vi "FGV ErrorLog.vi"(2 "Action":enum16{"Reset", "Enqueue", "Dequeue"}(ring), 3 "String to log":string) -> (1 "Logging":string[](array[string]))   [LabVIEW 2020, in "WSsupport.lvlib"]
uses:
  WSsupport.lvlib
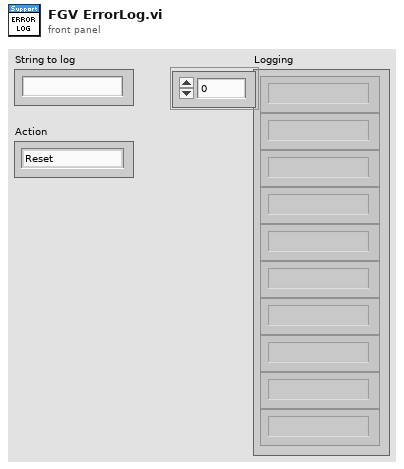
[diagram p1: front panel]
types:
  T1 = enum16{"open", "replace", "create", "open or create", "replace or create", "replace or create with confirmation"}
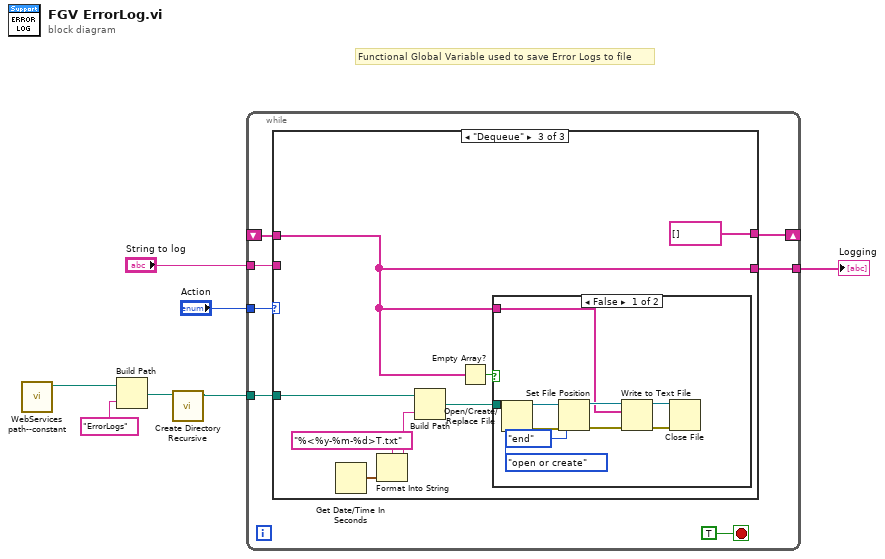
[diagram p0: block diagram]
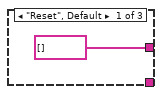
[diagram p2: hidden frame]
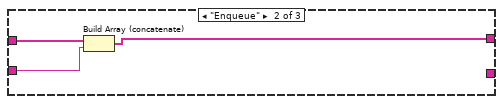
[diagram p3: hidden frame]
diagram:
  # "Functional Global Variable used to save Error Logs to file"
  n1 = call "WebServices path--constant.vi"() -> ("WebServices path"=w1:path)  [unwired: 11 in]
  n2 = Build Path(base path=w1, name or relative path="ErrorLogs") -> (appended path=w3:path)
  n3 = call <vilib>:"Create Directory Recursive.vi"("directory"=w3) -> ("directory copy"=w2:path)  [unwired: 4 in, 2 out]
  n4 = while {
    shift-right: [w12] -> _
    shift-left: _ -> [w11]
    tunnel: "Action" -> [w13]
    tunnel: "String to log" -> [w10]
    tunnel: [w9] -> w5
    tunnel: w2 -> [w8]
    stop <- TRUE stop-if-true
    n5 = case shown="\"Dequeue\"" w13 {
      tunnel: [string[] [] w16 string[] []] -> w12
      tunnel: w11 -> [_ w18 w20]
      tunnel: w10 -> [_ w17 _]
      tunnel: [_ _ w20] -> w9
      tunnel: w8 -> [_ _ w19]
      frame "Reset", Default {
      }
      frame "Enqueue" {
        n6 = Build Array (concatenate)(w18, w17) -> (w16:string[])
      }
      frame "Dequeue" {
        n7 = Get Date/Time In Seconds() -> (seconds since 1Jan1904=w25:timestamp)
        n8 = Format Into String(format string="%<%y-%m-%d>T.txt", w25) -> (resulting string=w23:string)  [unwired: 2 in, 1 out]
        n9 = Build Path(base path=w19, name or relative path=w23) -> (appended path=w22:path)
        n10 = Empty Array?(array=w20) -> (empty?=w21:bool)
        n11 = case shown="False" w21 {
          tunnel: w22 -> [w36 _]
          tunnel: w20 -> [w27 _]
          frame False {
            n12 = Open/Create/Replace File(file path (use dialog)=w36, operation (0:open)=T1."open or create") -> (refnum out=w34:refnum<file>, error out=w33:errorcluster)  [unwired: 4 in, 1 out]
            n13 = Set File Position(refnum=w34, from (0:start)=enum16{"start", "end", "current"}."end", error in=w33) -> (refnum out=w31:refnum<file>, error out=w30:errorcluster)  [unwired: 1 in]
            n14 = Write to Text File(file (use dialog)=w31, text=w27, error in=w30) -> (refnum out=w29:refnum<file>, error out=w28:errorcluster)  [unwired: 1 in, 1 out]
            n15 = Close File(refnum=w29, error in=w28) -> ()  [unwired: 2 out]
          }
          frame True {
          }
        }
      }
    }
  }
  "Logging" <- w5
